vi "read_params.vi"(8 "error in (no error)":errorcluster, 11 "MultiTaskElasticNetCV in":refnum<class "MultiTaskElasticNetCV.lvclass">) -> (0 "error out":errorcluster, 2 "params":T1={"l1_ratio"={"l1_ratio_type"="float", "l1_ratio_float"=0.5, "l1_ratio_list"=[]}, "eps"=0.001, "n_alphas"=100.0, "alphas"={"alphas_type"="None", "alphas_list"=[]}, "fit_intercept"=TRUE, "normalize"=FALSE, "max_iter"=1000.0, "tol"=0.0001, "cv"=5.0, "copy_X"=TRUE, "verbose"={"verbose_type"="int", "verbose_int"=0.0, "verbose_bool"=FALSE}, "n_jobs"=1.0, "random_state"=0.0, "selection"="cyclic"}, 3 "MultiTaskElasticNetCV out":refnum<class "MultiTaskElasticNetCV.lvclass">)   [LabVIEW 2020, in "MultiTaskElasticNetCV.lvclass"]
uses:
  MultiTaskElasticNetCV.lvclass
  Controls/multi_task_elasticnet_cv_params.ctl
  MultiTaskElasticNetCV.lvclass/MultiTaskElasticNetCV.ctl
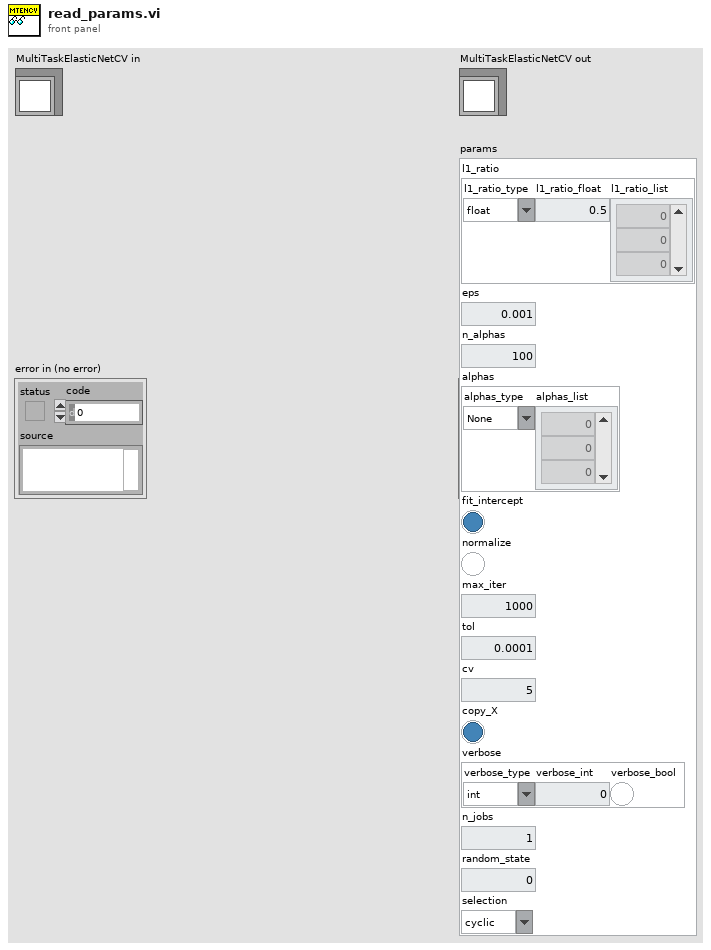
[diagram p1: front panel]
types:
  T1 = typedef "multi_task_elasticnet_cv_params.ctl" = cluster{"l1_ratio":cluster{"l1_ratio_type":string, "l1_ratio_float":dbl, "l1_ratio_list":dbl[]}, "eps":dbl, "n_alphas":dbl, "alphas":cluster{"alphas_type":string, "alphas_list":dbl[]}, "fit_intercept":bool, "normalize":bool, "max_iter":dbl, "tol":dbl, "cv":dbl, "copy_X":bool, "verbose":cluster{"verbose_type":string, "verbose_int":dbl, "verbose_bool":bool}, "n_jobs":dbl, "random_state":dbl, "selection":string}
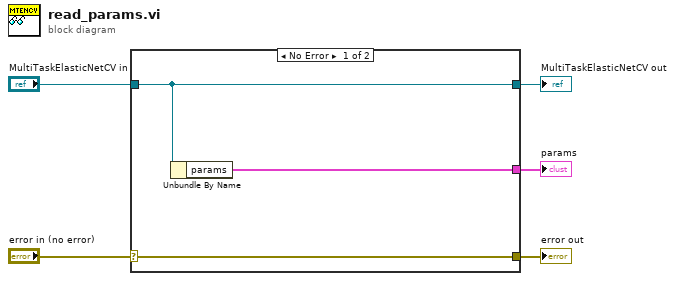
[diagram p0: block diagram]
diagram:
  n1 = case shown="No Error" "error in (no error)" {
    selector: "error in (no error)" -> [w8 w9]
    tunnel: [w8 w9] -> w4
    tunnel: [w7 w10] -> w2
    tunnel: "MultiTaskElasticNetCV in" -> [w7 w10]
    tunnel: [w6 _] -> w1
    frame No Error {
      n2 = Unbundle By Name(w7) -> ("params"=w6:T1)
    }
    frame Error {
    }
  }
  "error out" <- w4
  "MultiTaskElasticNetCV out" <- w2
  "params" <- w1
